vi "SignalGenerator.vi"(4 "Frequency":dbl, 5 "Amplitude":dbl) -> ()   [LabVIEW 2014]
panel:
  in  "error in (no error)":errorcluster
  out "error out":errorcluster
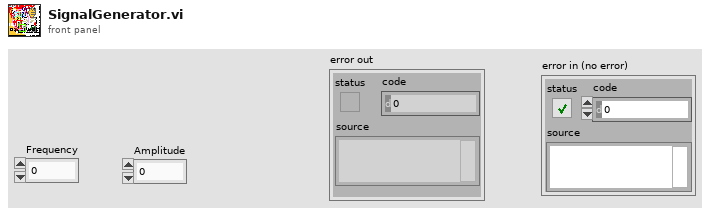
[diagram p1: front panel]
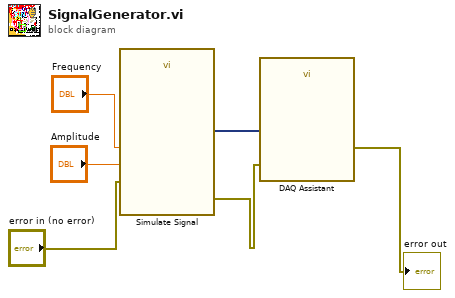
[diagram p0: block diagram]
diagram:
  n1 = call "Simulate Signal"("Frequency"="Frequency", "Amplitude"="Amplitude", "error in (no error)"="error in (no error)") -> ("Sine"=w4:dynamicdata, "error out"=w6:errorcluster)  [unwired: 11 in]
  n2 = call "DAQ Assistant"("data"=w4, "error in"=w6) -> ("error out"=→"error out":errorcluster)  [unwired: 16 in, 1 out]
